vi "Main.vi"(11 "Module Admin":refnum<class "Delacor_lib_QMH_Module Admin.lvclass">) -> ()   [LabVIEW 2019, in "Camera.lvlib"]
doc: "This template is based off of the Queued Message Handler design pattern and the Queued Message Handler project template that ships with LabVIEW.\n\nThe main difference is that the queue is private to this module and communication between modules is performed via Broadcast and Request events.\n\nRequest events are wrapped in public API methods and are handled in the Event Handling Loop (EHL) of this VI. Any module can register for Broadcast events sent by this module. The EHL generates messages based on user interface actions.\n\nThe Message Handling Loop (MHL) processes messages generated by the EHL, or by other messages. The messages are string values, so new messages can be added easily to the Message Cases case structure in the MHL. Each message cluster can also provide an optional value for Message Data, which is a variant that can be converted to whatever message-specific data is required.\n_____\nBased on Delacor QMH Project Template 5.0.0.82."
uses:
  Camera.lvlib
  <vilib>/Delacor/Delacor QMH/Libraries/Module Admin_class/Delacor_lib_QMH_Module Admin.lvclass
  Module Data--cluster.ctl
  <vilib>/Delacor/Delacor QMH/Libraries/Message Queue_class/Delacor_lib_QMH_Message Queue.lvclass/Delacor_lib_QMH_Message Queue.ctl
  Stop Argument--cluster.ctl
  <vilib>/Delacor/Delacor QMH/Libraries/Module Admin_class/Delacor_lib_QMH_Module Admin.lvclass/Delacor_lib_QMH_Module Admin.ctl
  Get Image Argument--cluster.ctl
  Get Image (Reply Payload)--cluster.ctl
  <vilib>/Utility/miscctls.llb/LVPointTypeDef.ctl
  <vilib>/Delacor/Delacor QMH/Libraries/Message Queue_class/Delacor_lib_QMH_Enqueue Message (Single).vi
  <vilib>/Delacor/Delacor QMH/Libraries/Module Admin_class/Delacor_lib_QMH_Get External Launch.vi
  <vilib>/numeric/Random Number (Range) U64.vi
  <vilib>/numeric/sub_Random U32.vi
  <vilib>/Utility/error.llb/Error Cluster From Error Code.vi
  <vilib>/ErrorRing/Error Ring.xnode
  <vilib>/Delacor/Delacor QMH/Libraries/Message Queue_class/Delacor_lib_QMH_Message Queue.lvclass
panel:
  in  "Simulate MHL Error":bool
  in  "Simulate EHL Error":bool
  out "error out":errorcluster
  out "Status":string
  # "PICam Device"
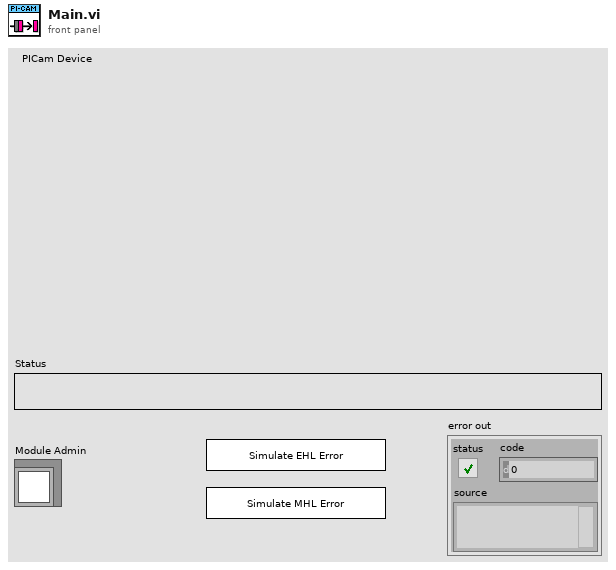
[diagram p1: front panel]
types:
  T1 = typedef "Camera.lvlib/Request Events--cluster.ctl" = cluster{"Stop Module":refnum<user-event>, "Show Panel":refnum<user-event>, "Hide Panel":refnum<user-event>, "Get Module Execution Status":refnum<user-event>, "Show Diagram":refnum<user-event>, "Get Image":refnum<user-event>}
  T2 = typedef "Camera.lvlib/Module Data--cluster.ctl" = cluster{"Status":string}
  T3 = enum32{"invalid lock state", "Not Locked", "Locked (No Password)", "Password-protected"}
  T4 = typedef "Camera.lvlib/Stop Argument--cluster.ctl" = cluster{"Origin":string, "Exit via Stop Module Req?":bool, "Wait for Module to stop?":bool}
  T5 = typedef "Camera.lvlib/Get Image Argument--cluster.ctl" = cluster{"Wait Notifier":refnum<notifier>, "wait for reply":bool}
  T6 = typedef "LVPointTypeDef.ctl" = cluster{"Horizontal":i16, "Vertical":i16}
  T7 = enum32{"Invalid", "Standard", "Closed", "Hidden", "Minimized", "Maximized"}
  T8 = typedef "Camera.lvlib/Get Image (Reply Payload)--cluster.ctl" = cluster{"Image":u16[][], "Get Image_error":errorcluster}
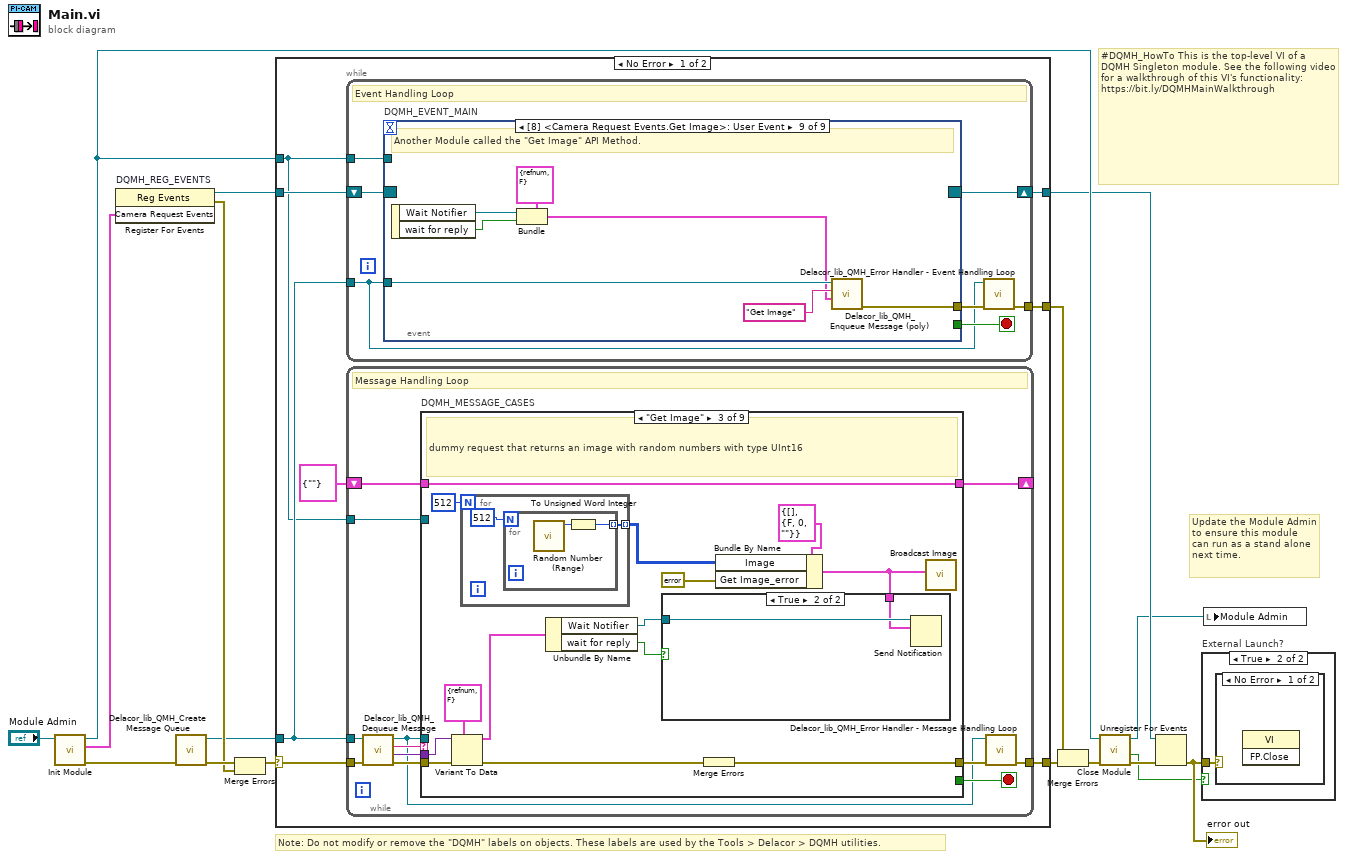
[diagram p0: block diagram]
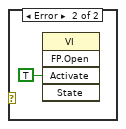
[diagram p3: hidden frame]
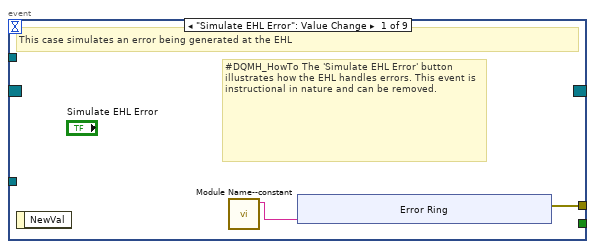
[diagram p4: hidden frame]
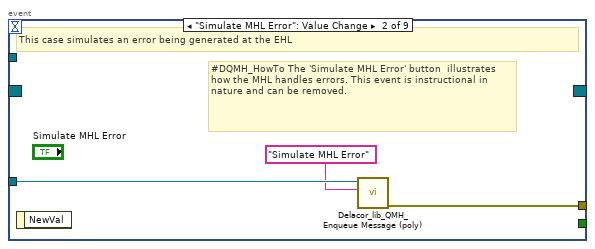
[diagram p5: hidden frame]
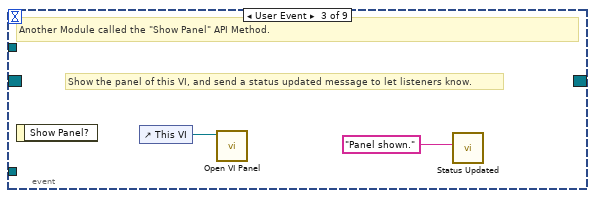
[diagram p6: hidden frame]
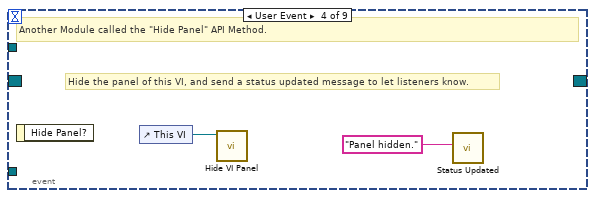
[diagram p7: hidden frame]
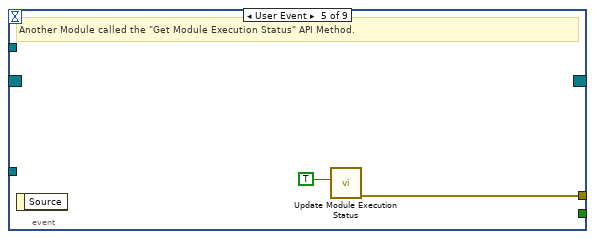
[diagram p8: hidden frame]
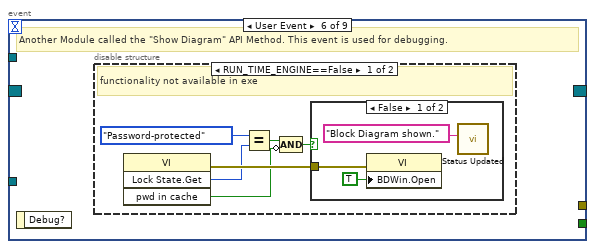
[diagram p9: hidden frame]
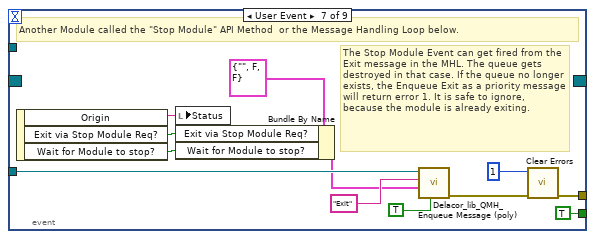
[diagram p12: hidden frame]
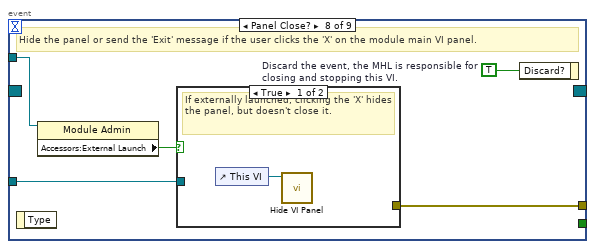
[diagram p13: hidden frame]
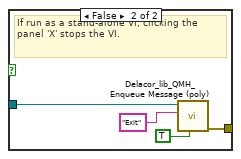
[diagram p14: hidden frame]
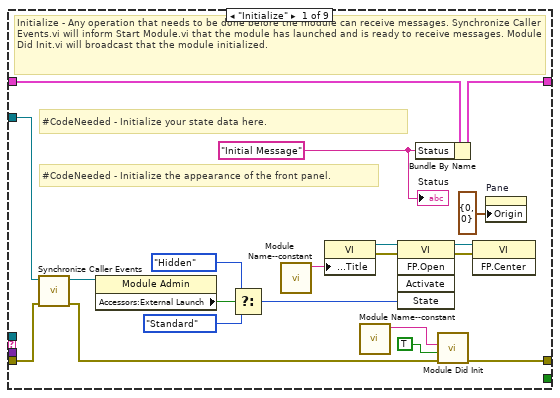
[diagram p15: hidden frame]
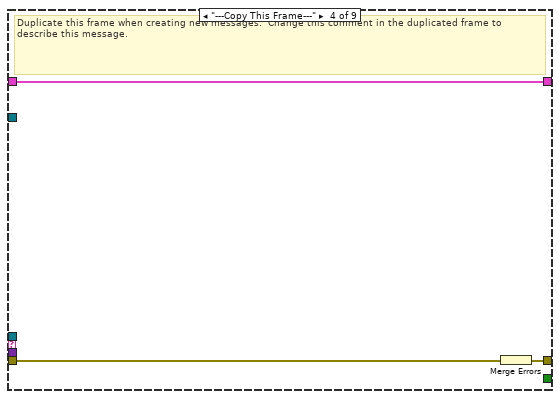
[diagram p18: hidden frame]
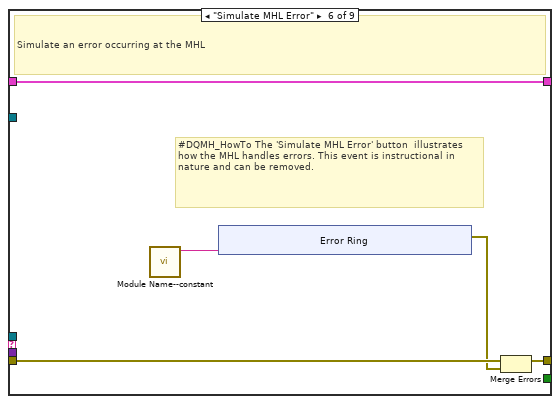
[diagram p20: hidden frame]
diagram:
  # "#DQMH_HowTo This is the top-level VI of a DQMH Singleton module. See the following video for a walkthrough of this VI's functionality: https://bit.ly/DQMHMainWalkthrough"
  # "Note: Do not modify or remove the \"DQMH\" labels on objects. These labels are used by the Tools > Delacor > DQMH utilities."
  # "Update the Module Admin to ensure this module can run as a stand alone next time."
  n1 = call "Init Module.vi"("Singleton Module Admin in"="Module Admin") -> ("error out"=w16:errorcluster, "Camera Request Events"=w5:T1, "Singleton Module Admin out"=w8:refnum<class "Delacor_lib_QMH_Module Admin.lvclass">)  [unwired: 8 in]
  n2 = register-events "DQMH_REG_EVENTS"(w5) -> (reference out=w6:refnum<event-registration>, error out=w9:errorcluster)  [unwired: 2 in]
  n3 = call <vilib>:"Delacor_lib_QMH_Create Message Queue.vi"("error in (no error)"=w16) -> ("error out"=w11:errorcluster, "Message Queue"=w4:refnum<class "Delacor_lib_QMH_Message Queue.lvclass">)  [unwired: 9 in]
  n4 = Merge Errors(w11, w9) -> (w10:errorcluster)
  n5 = case shown="No Error" w10 {
    selector: w10 -> [w23 w208]
    tunnel: [w25 w207] -> w17
    tunnel: [w22 w213] -> w7
    tunnel: w6 -> [w20 w213]
    tunnel: w4 -> [w19 w206]
    tunnel: [w24 _] -> w14
    tunnel: w8 -> [w18 w209]
    frame No Error {
      n6 = while {
        tunnel: w19 -> [w26]
        shift-right: [w29] -> w22
        shift-left: w20 -> [w30]
        tunnel: [w31] -> w24
        tunnel: w18 -> [w27]
        stop <- w28 stop-if-true
        # "Event Handling Loop"
        n7 = event "DQMH_EVENT_MAIN" shown="[8] <Camera Request Events.Get Image>: User Event" {
          selector: w30 -> [_ _ _ _ _ _ _ _ _]
          dyn-events: [_ _ _ _ _ _ _ _ _] -> w29
          timeout: _ -> [_ _ _ _ _ _ _ _ _]
          tunnel: [_ _ _ _ _ _ TRUE ("Discard?") _ _] -> w28
          tunnel: w26 -> [_ w43 _ _ _ _ w67 w74 w88]
          tunnel: [w34 w44 _ _ w50 _ w70 w76 w82] -> w32
          tunnel: w27 -> [_ _ _ _ _ _ _ w73 _]
          event "Simulate EHL Error": Value Change {
            # "#DQMH_HowTo The 'Simulate EHL Error' button  illustrates how the EHL handles errors. This event is instructional in nature and can be removed."
            # "This case simulates an error being generated at the EHL"
            n8 = event-data() -> ()  [unwired: 1 in, 1 out]
            n9 = call "Module Name--constant.vi"() -> ("Module Name"=w33:string)  [unwired: 11 in]
            n10 = xnode "Error Ring"("parameter 0"=w33) -> ("error out"=w34:errorcluster)
          }
          event "Simulate MHL Error": Value Change {
            # "#DQMH_HowTo The 'Simulate MHL Error' button  illustrates how the MHL handles errors. This event is instructional in nature and can be removed."
            # "This case simulates an error being generated at the EHL"
            n11 = event-data() -> ()  [unwired: 1 in, 1 out]
            n12 = call-poly <vilib>:"Delacor_lib_QMH_Enqueue Message (poly).vi"("Message"="Simulate MHL Error", "Message Queue in"=w43) -> ("error out"=w44:errorcluster)  [unwired: 8 in, 1 out]
          }
          event User Event {
            # "Show the panel of this VI, and send a status updated message to let listeners know."
            # "Another Module called the \"Show Panel\" API Method."
            n13 = event-data() -> ()  [unwired: 1 in, 1 out]
            n14 = control-ref of="This VI"() -> (w46:refnum<vi>)
            n15 = call "Open VI Panel.vi"("VI"=w46) -> ()  [unwired: 10 in, 1 out]
            n16 = call "Status Updated.vi"("Status"="Panel shown." ("format string")) -> ()  [unwired: 10 in, 1 out]
          }
          event User Event {
            # "Hide the panel of this VI, and send a status updated message to let listeners know."
            # "Another Module called the \"Hide Panel\" API Method."
            n17 = event-data() -> ()  [unwired: 1 in, 1 out]
            n18 = control-ref of="This VI"() -> (w48:refnum<vi>)
            n19 = call "Hide VI Panel.vi"("VI"=w48) -> ()  [unwired: 10 in, 1 out]
            n20 = call "Status Updated.vi"("Status"="Panel hidden." ("format string")) -> ()  [unwired: 10 in, 1 out]
          }
          event User Event {
            # "Another Module called the \"Get Module Execution Status\" API Method."
            n21 = event-data() -> ()  [unwired: 1 in, 1 out]
            n22 = call "Update Module Execution Status.vi"("Running?"=TRUE) -> ("error out"=w50:errorcluster)  [unwired: 10 in]
          }
          event User Event {
            # "Another Module called the \"Show Diagram\" API Method. This event is used for debugging."
            n23 = event-data() -> ()  [unwired: 1 in, 1 out]
            n24 = disable-structure shown="RUN_TIME_ENGINE==False" {
              frame condition #0 (active) {
                # "functionality not available in exe"
                n25 = invoke class="VI" method="Lock State.Get"() -> (error out=w56:errorcluster, "Get Lock State"=w55:T3, "pwd in cache"=w52:bool)  [unwired: 4 in, 1 out]
                n26 = Equal?(x=T3."Password-protected", y=w55) -> (x = y?=w53:bool)
                n27 = Compound Arithmetic op=AND(w53, invert w52) -> (w51:bool)
                n28 = case shown="False" w51 {
                  tunnel: w56 -> [w59 _]
                  frame False {
                    n29 = property class="VI"(error in=w59, "BDWin.Open"=TRUE ("Block Diagram Window:Open")) -> ()  [unwired: 1 in, 2 out]
                    n30 = call "Status Updated.vi"("Status"="Block Diagram shown." ("format string")) -> ()  [unwired: 10 in, 1 out]
                  }
                  frame True {
                    # "Password-protected VI, and the password is not in the cache. Do not show the diagram."
                  }
                }
              }
              frame condition #1 {
              }
            }
          }
          event User Event {
            # "The Stop Module Event can get fired from the Exit message in the MHL. The queue gets destroyed in that case. If the queue no longer exists, the Enqueue Exit as a priority message will return error 1. It is safe to ignore, because the module is already exiting."
            # "Another Module called the \"Stop Module\" API Method  or the Message Handling Loop below."
            n31 = event-data() -> ("Origin"=w66:string, "Exit via Stop Module Req?"=w62:bool, "Wait for Module to stop?"=w61:bool)  [unwired: 1 in]
            n32 = local write "Status"(w66) -> ()
            n33 = Bundle By Name(cluster=T4 {"Origin"="", "Exit via Stop Module Req?"=FALSE, "Wait for Module to stop?"=FALSE} ("Stop Argument"), "Exit via Stop Module Req?"=w62, "Wait for Module to stop?"=w61) -> (w60:T4)
            n34 = call-poly <vilib>:"Delacor_lib_QMH_Enqueue Message (poly).vi"("Priority Message? (F)"=TRUE, "Message Data"=w60, "Message"="Exit", "Message Queue in"=w67) -> ("error out"=w71:errorcluster)  [unwired: 6 in, 1 out]
            n35 = call <vilib>:"Clear Errors.vi"("error in (no error)"=w71, "specific error code to clear (0: all)"=1) -> ("error out"=w70:errorcluster)  [unwired: 4 in, 1 out]
          }
          event Panel Close? {
            w75 = TRUE  # Discard the event, the MHL is responsible for closing and stopping this VI.
            # "Hide the panel or send the 'Exit' message if the user clicks the 'X' on the module main VI panel."
            n36 = event-data() -> ()  [unwired: 1 in, 1 out]
            n37 = property class="Module Admin"(reference=w73) -> ("Accessors:External Launch"=w72:bool)  [unwired: 1 in, 2 out]
            n38 = case shown="True" w72 {
              tunnel: w74 -> [_ w80]
              tunnel: [_ w81] -> w76
              frame True {
                # "If externally launched, clicking the 'X' hides the panel, but doesn't close it."
                n39 = control-ref of="This VI"() -> (w77:refnum<vi>)
                n40 = call "Hide VI Panel.vi"("VI"=w77) -> ()  [unwired: 10 in, 1 out]
              }
              frame False {
                # "If run as a stand-alone VI, clicking the panel 'X' stops the VI."
                n41 = call-poly <vilib>:"Delacor_lib_QMH_Enqueue Message (poly).vi"("Priority Message? (F)"=TRUE, "Message"="Exit", "Message Queue in"=w80) -> ("error out"=w81:errorcluster)  [unwired: 7 in, 1 out]
              }
            }
            n42 = event-data("Discard?"=w75) -> ()  [unwired: 1 in, 1 out]
          }
          event User Event {
            # "Another Module called the \"Get Image\" API Method."
            n43 = event-data() -> ("Wait Notifier"=w84:refnum<notifier>, "wait for reply"=w83:bool)  [unwired: 1 in]
            n44 = Bundle(cluster=T5 {"Wait Notifier"=refnum, "wait for reply"=FALSE} ("Get Image Argument"), "Wait Notifier"=w84, "wait for reply"=w83) -> (w85:T5)
            n45 = call-poly <vilib>:"Delacor_lib_QMH_Enqueue Message (poly).vi"("Message Data"=w85, "Message"="Get Image", "Message Queue in"=w88) -> ("error out"=w82:errorcluster)  [unwired: 7 in, 1 out]
          }
        }
        n46 = call-dynamic "Delacor_lib_QMH_Error Handler - Event Handling Loop.vi"("error in (no error)"=w32, "Message Queue in"=w26) -> ("dup error in"=w31:errorcluster)  [unwired: 8 in, 1 out]
      }
      n47 = while {
        tunnel: w19 -> [w91]
        shift-right: [w95] -> _
        shift-left: T2 {"Status"=""} ("Data Cluster") -> [w96]
        tunnel: w23 -> [w99]
        tunnel: [w97] -> w25
        tunnel: w18 -> [w89]
        stop <- w94 stop-if-true
        # "Message Handling Loop"
        n48 = call-dynamic "Delacor_lib_QMH_Dequeue Message.vi"("error in (no error)"=w99, "Message Queue in"=w91) -> ("error out"=w98:errorcluster, "Message Data"=w92:variant, "Message"=w93:string, "Message Queue out"=w90:refnum<class "Delacor_lib_QMH_Message Queue.lvclass">)  [unwired: 6 in]
        n49 = case "DQMH_MESSAGE_CASES" shown="\"Get Image\"" w93 {
          selector: w93 -> [_ _ _ _ _ _ _ _ w193]
          tunnel: w90 -> [_ _ _ _ _ _ w163 w185 _]
          tunnel: w98 -> [w118 w122 w136 w145 w147 w152 w170 w191 w195]
          tunnel: [w116 w122 w126 w144 w147 w151 w166 w188 w196] -> w100
          tunnel: w96 -> [w107 w121 w135 w143 w146 w149 w165 w184 w194]
          tunnel: [w106 w121 w135 w143 w146 w149 w165 w184 w194] -> w95
          tunnel: [_ _ _ _ _ _ _ w183 _] -> w94
          tunnel: w92 -> [_ _ w133 _ _ _ w164 w182 _]
          tunnel: w89 -> [w108 _ _ _ _ _ w162 w177 _]
          frame "Initialize" {
            w101 = "Initial Message" ("Initial Message")
            # "#CodeNeeded - Initialize the appearance of the front panel."
            # "#CodeNeeded - Initialize your state data here."
            # "Initialize - Any operation that needs to be done before the module can receive messages. Synchronize Caller Events.vi will inform Start Module.vi that the module has launched and is ready to receive messages. Module Did Init.vi will broadcast that the module initialized."
            n50 = call "Synchronize Caller Events.vi"("error in (no error)"=w118, "Singleton Module Admin in"=w108) -> ("error out"=w117:errorcluster, "Singleton Module Admin out"=w103:refnum<class "Delacor_lib_QMH_Module Admin.lvclass">)  [unwired: 8 in]
            n51 = property class="Module Admin"(reference=w103) -> ("Accessors:External Launch"=w112:bool)  [unwired: 1 in, 2 out]
            n52 = Select(t=T7."Hidden" ("State"), s=w112, f=T7."Standard" ("State")) -> (s? t:f=w109:T7)
            n53 = call "Module Name--constant.vi"() -> ("Module Name"=w115:string)  [unwired: 11 in]
            n54 = property class="VI"("Front Panel.Title"=w115) -> (reference out=w114:refnum<vi>, error out=w120:errorcluster)  [unwired: 2 in]
            n55 = call "Module Name--constant.vi"() -> ("Module Name"=w104:string)  [unwired: 11 in]
            n56 = invoke class="VI" method="FP.Open"(reference=w114, error in=w120, "State"=w109) -> (reference out=w113:refnum<vi>, error out=w119:errorcluster)  [unwired: 2 in, 3 out]
            n57 = Bundle By Name(cluster=w107, "Status"=w101) -> (w106:T2)
            n58 = call "Module Did Init.vi"("error in (no error)"=w117, "Initialized?"=TRUE, "Origin"=w104) -> ("error out"=w116:errorcluster)  [unwired: 8 in]
            n59 = invoke class="VI" method="FP.Center"(reference=w113, error in=w119) -> ()  [unwired: 1 in, 3 out]
            n60 = property on="Pane" class="Pane"("Origin"=T6 {"Horizontal"=0, "Vertical"=0}) -> ()  [unwired: 2 in, 2 out]
            "Status" <- w101
          }
          frame "--- Module Specific ---" {
            # "Separator -- The following cases handle messages specific to this Module."
          }
          frame "Get Image" {
            # "dummy request that returns an image with random numbers with type UInt16"
            n61 = Variant To Data(error in=w136, type=T5 {"Wait Notifier"=refnum, "wait for reply"=FALSE} ("Get Image Argument"), Variant=w133) -> (data=w131:T5, error out=w134:errorcluster)
            n62 = for {
              N: 512 -> [_]
              tunnel: [w138] -> w124 mode=indexing
              n63 = for {
                N: 512 -> [_]
                tunnel: [w139] -> w138 mode=indexing
                n64 = call-poly <vilib>:"Random Number (Range).vi"() -> ("number"=w140:u64)  [unwired: 11 in]
                n65 = To Unsigned Word Integer(number=w140) -> (unsigned 16bit integer=w139:u16)
              }
            }
            n66 = Unbundle By Name(w131) -> ("Wait Notifier"=w130:refnum<notifier>, "wait for reply"=w129:bool)
            n67 = Merge Errors(w134) -> (w126:errorcluster)
            n68 = Bundle By Name(cluster=T8 {"Image"=[], "Get Image_error"={"status"=FALSE, "code"=0, "source"=""}} ("Get Image (Reply Payload)"), "Image"=w124, "Get Image_error"=errorcluster {"status"=FALSE, "code"=0, "source"=""}) -> (w128:T8)
            n69 = case shown="True" w129 {
              tunnel: w130 -> [_ w142]
              tunnel: w128 -> [_ w141]
              frame False {
              }
              frame True {
                n70 = Send Notification(notification=w141, notifier=w142) -> ()  [unwired: 1 in, 2 out]
              }
            }
            n71 = call "Broadcast Image.vi"("Reply Payload"=w128) -> ()  [unwired: 10 in, 1 out]
          }
          frame "---Copy This Frame---" {
            # "Duplicate this frame when creating new messages.  Change this comment in the duplicated frame to describe this message."
            n72 = Merge Errors(w145) -> (w144:errorcluster)
          }
          frame "--- Exit and Error Handling---" {
            # "Separator - The following cases handle errors and exit messages."
          }
          frame "Simulate MHL Error" {
            # "#DQMH_HowTo The 'Simulate MHL Error' button  illustrates how the MHL handles errors. This event is instructional in nature and can be removed."
            # "Simulate an error occurring at the MHL"
            n73 = call "Module Name--constant.vi"() -> ("Module Name"=w148:string)  [unwired: 11 in]
            n74 = xnode "Error Ring"("parameter 0"=w148) -> ("error out"=w150:errorcluster)
            n75 = Merge Errors(w152, w150) -> (w151:errorcluster)
          }
          frame "Error" {
            # "#CodeRecommended - If you ever change the name of this \"Error\" message, you'll need to update the name in the Check Loop Error.vi as well."
            # "#CodeRecommended - If the module is running in standalone mode (External Launch = FALSE), this code will pop up an error dialog and call the 'Exit' message if an error occurs. Add more fine-grained error handling here."
            # "Error - Check the error message data and respond accordingly. This message is sent by the \"Error Handler\" VIs at the end of each loop in this application."
            n76 = property class="Module Admin"(reference=w162) -> ("Accessors:External Launch"=w161:bool)  [unwired: 1 in, 2 out]
            n77 = Variant To Data(error in=w170, type=errorcluster {"status"=FALSE, "code"=0, "source"=""} ("error constant"), Variant=w164) -> (data=w171:errorcluster, error out=w168:errorcluster)
            n78 = call "Module Name--constant.vi"() -> ("Module Name"=w160:string)  [unwired: 11 in]
            n79 = call "Error Reported.vi"("Additional Information"=w160, "Error"=w171) -> ()  [unwired: 9 in, 1 out]
            n80 = case shown="False" w161 {
              tunnel: [w176 _] -> w167
              tunnel: w163 -> [w174 _]
              tunnel: w171 -> [w175 _]
              frame False {
                # "If the module is running standalone, then pop up an error dialog and call the \"Exit\" message."
                n81 = call <vilib>:"Simple Error Handler.vi"("error in (no error)"=w175) -> ()  [unwired: 4 in, 5 out]
                n82 = call-poly <vilib>:"Delacor_lib_QMH_Enqueue Message (poly).vi"("Priority Message? (F)"=TRUE, "Message"="Exit", "Message Queue in"=w174) -> ("error out"=w176:errorcluster)  [unwired: 7 in, 1 out]
              }
              frame True {
                # "If the module was launched externally, calling the Error Reported broadcast VI is the only action performed by the \"Error\" message. The module's caller can then process the error appropriately."
              }
            }
            n83 = Merge Errors(w168, w167) -> (w166:errorcluster)
            n84 = local write "error out"(w166) -> ()
          }
          frame "Exit" {
            w181 = 91  # 91: not all Exit messages will have an argument
            w183 = TRUE  # Stop the VI
            # "Release the message queue reference"
            # "#CodeNeeded - Add any required cleanup code here"
            # "Exit - Exit the application."
            n85 = Variant To Data(error in=w191, type=T4 {"Origin"="", "Exit via Stop Module Req?"=FALSE, "Wait for Module to stop?"=FALSE} ("Stop Argument"), Variant=w182) -> (data=w179:T4, error out=w187:errorcluster)
            n86 = call <vilib>:"Clear Errors.vi"("error in (no error)"=w187, "specific error code to clear (0: all)"=w181) -> ("error out"=w190:errorcluster)  [unwired: 4 in, 1 out]
            n87 = control-ref of="This VI"() -> (w178:refnum<vi>)
            n88 = call-dynamic "Delacor_lib_QMH_Release Message Queue.vi"("error in (no error)"=w190, "Message Queue"=w185) -> ("error out"=w189:errorcluster)  [unwired: 9 in]
            n89 = call "Handle Exit.vi"("Stop Argument"=w179, "Admin in"=w177, "VI reference"=w178) -> ("error out"=w186:errorcluster)  [unwired: 7 in, 1 out]
            n90 = Merge Errors(w189, w186) -> (w188:errorcluster)
          }
          frame Default {
            # "'Default' case only runs if there is a message that isn't defined in any of the other cases.  Output a programming error."
            n91 = call "Module Name--constant.vi"() -> ("Module Name"=w192:string)  [unwired: 11 in]
            n92 = xnode "Error Ring"("parameter 0"=w193, "parameter 1"=w192) -> ("error out"=w197:errorcluster)
            n93 = Merge Errors(w195, w197) -> (w196:errorcluster)
          }
        }
        n94 = call-dynamic "Delacor_lib_QMH_Error Handler - Message Handling Loop.vi"("error in (no error)"=w100, "Message Queue in"=w90) -> ("dup error in"=w97:errorcluster)  [unwired: 8 in, 1 out]
      }
    }
    frame Error {
      # "Synchronize Caller Events.vi will inform Start Module.vi that the module has launched and will let the code calling Start Module.vi register for broadcasts and would permit the caller receive the broadcast that an error occurred at launch time."
      n95 = call-dynamic "Delacor_lib_QMH_Release Message Queue.vi"("error in (no error)"=w208, "Message Queue"=w206) -> ("error out"=w207:errorcluster)  [unwired: 9 in]
      n96 = call "Synchronize Caller Events.vi"("Singleton Module Admin in"=w209) -> ("error out"=w214:errorcluster)  [unwired: 9 in, 1 out]
      n97 = call "Module Name--constant.vi"() -> ("Module Name"=w212:string)  [unwired: 11 in]
      n98 = Format Into String(format string="An error occurred during initialization. %s is no longer running.", w212) -> (resulting string=w210:string)  [unwired: 2 in, 1 out]
      n99 = Merge Errors(w207, w214) -> (w215:errorcluster)
      n100 = call "Error Reported.vi"("Additional Information"=w210, "Error"=w215) -> ()  [unwired: 9 in, 1 out]
    }
  }
  n101 = Merge Errors(w14, w17) -> (w13:errorcluster)
  n102 = call "Close Module.vi"("error in (no error)"=w13, "Module Admin in"=w8) -> ("error out"=w15:errorcluster, "External Launch"=w1:bool, "Module Admin out"=w2:refnum<class "Delacor_lib_QMH_Module Admin.lvclass">)  [unwired: 7 in]
  n103 = Unregister For Events(event registration refnum=w7, error in=w15) -> (error out=w12:errorcluster)
  "error out" <- w12
  n104 = case "External Launch?" shown="True" w1 {
    tunnel: w12 -> [_ w216]
    frame False {
    }
    frame True {
      n105 = case shown="No Error" w216 {
        frame No Error {
          n106 = invoke class="VI" method="FP.Close"() -> ()  [unwired: 3 in, 3 out]
        }
        frame Error {
          n107 = invoke class="VI" method="FP.Open"("Activate"=TRUE ("Activate?")) -> ()  [unwired: 4 in, 5 out]
        }
      }
    }
  }
  n108 = local write "Module Admin"(w2) -> ()
